vi "AB_RW_Project_Source_Library.vi"(7 "action":T3, 8 "error in (no error)":errorcluster, 9 "index in":i32, 10 "dataSource in":T2, 11 "buildObject":T1) -> (0 "error out":errorcluster, 1 "index out":i32, 2 "dataSource out":T2, 3 "buildObject out":T1)   [LabVIEW 2020]
doc: "Reads and writes the data to the object property bag."
uses:
  <resource>/Framework/Providers/API/ItemRef.ctl
  <vilib>/AppBuilder/RW_Project/AB_RW_Project_Source_Library_Data.ctl
  <vilib>/AppBuilder/RW_Project/AB_RW_Project_PropBag_Action.ctl
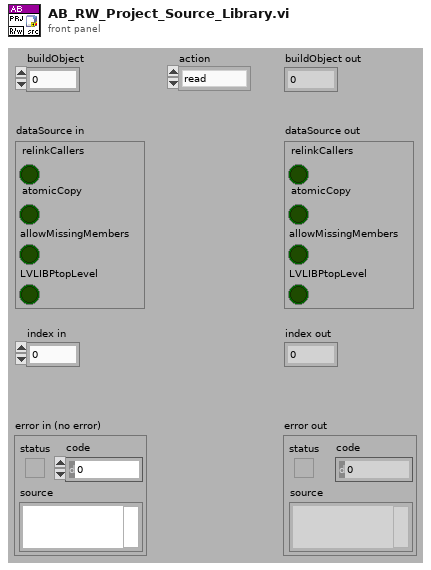
[diagram p1: front panel]
types:
  T1 = typedef "ItemRef.ctl" = u64
  T2 = typedef "AB_RW_Project_Source_Library_Data.ctl" = cluster{"relinkCallers":bool, "atomicCopy":bool, "allowMissingMembers":bool, "LVLIBPtopLevel":bool}
  T3 = typedef "AB_RW_Project_PropBag_Action.ctl" = enum16{"read", "write", "clear", "readPrevious", "writePrevious", "clearPrevious"}
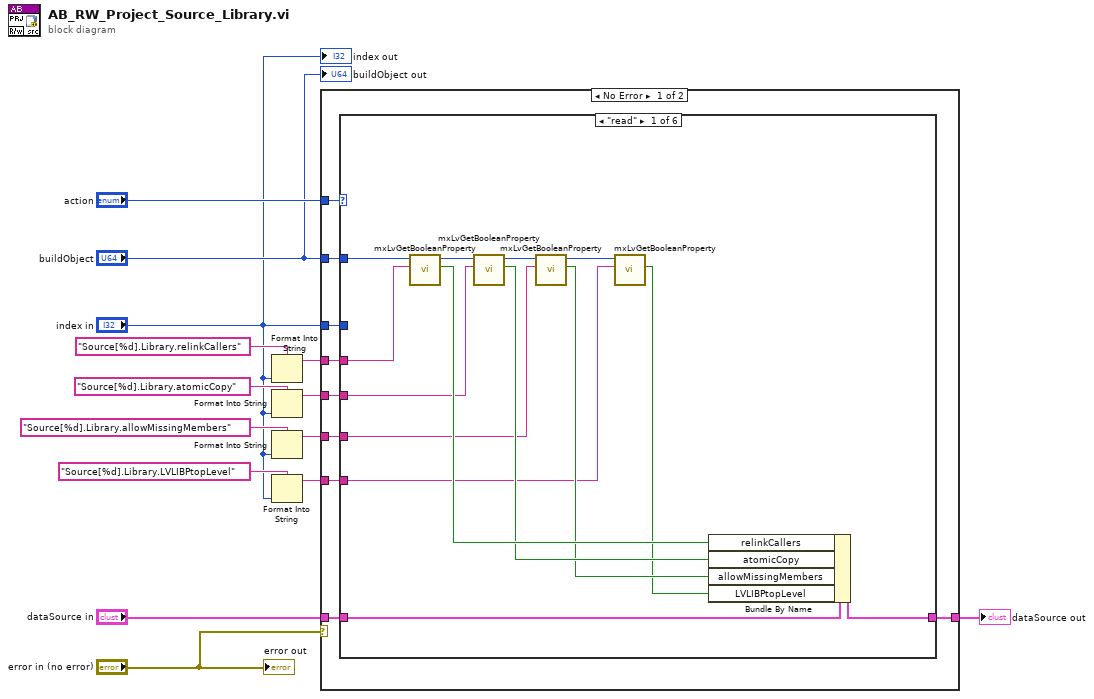
[diagram p0: block diagram]
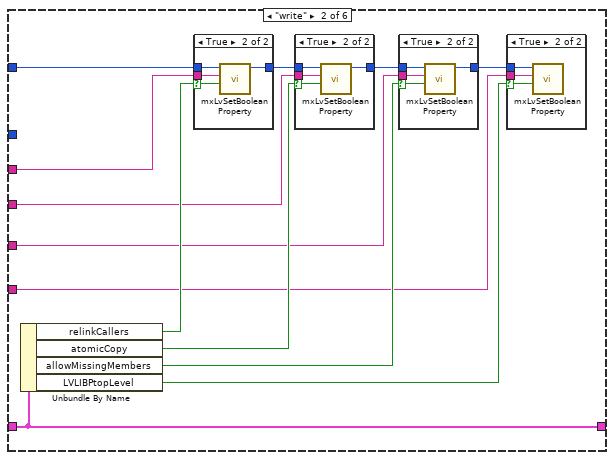
[diagram p2: hidden frame]
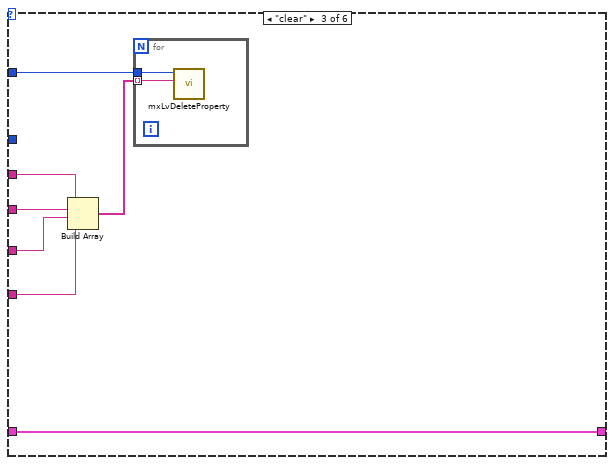
[diagram p7: hidden frame]
diagram:
  n1 = Format Into String(format string="Source[%d].Library.relinkCallers", "index in") -> (resulting string=w11:string)  [unwired: 2 in, 1 out]
  n2 = Format Into String(format string="Source[%d].Library.atomicCopy", "index in") -> (resulting string=w9:string)  [unwired: 2 in, 1 out]
  n3 = Format Into String(format string="Source[%d].Library.allowMissingMembers", "index in") -> (resulting string=w4:string)  [unwired: 2 in, 1 out]
  n4 = Format Into String(format string="Source[%d].Library.LVLIBPtopLevel", "index in") -> (resulting string=w1:string)  [unwired: 2 in, 1 out]
  n5 = case shown="No Error" "error in (no error)" {
    tunnel: "action" -> [w23 _]
    tunnel: "dataSource in" -> [w22 w81]
    tunnel: w11 -> [w21 _]
    tunnel: w9 -> [w20 _]
    tunnel: "index in" -> [w19 _]
    tunnel: [w18 w81] -> w8
    tunnel: "buildObject" -> [w17 _]
    tunnel: w4 -> [w16 _]
    tunnel: w1 -> [w15 _]
    frame No Error {
      n6 = case shown="\"read\"" w23 {
        tunnel: w17 -> [w35 w49 w71 _ _ _]
        tunnel: w22 -> [w37 w50 w75 w78 w79 w80]
        tunnel: w21 -> [w33 w47 w74 _ _ _]
        tunnel: w20 -> [w31 w45 w73 _ _ _]
        tunnel: w19 -> [_ _ _ _ _ _]
        tunnel: [w36 w50 w75 w78 w79 w80] -> w18
        tunnel: w16 -> [w29 w42 w70 _ _ _]
        tunnel: w15 -> [w25 w39 w69 _ _ _]
        frame "read" {
          n7 = call <resource>:"mxLvGetBooleanProperty.vi"("Tag"=w33, "Item"=w35) -> ("Value"=w34:bool, "Item"=w32:T1)  [unwired: 7 in, 1 out]
          n8 = call <resource>:"mxLvGetBooleanProperty.vi"("Tag"=w31, "Item"=w32) -> ("Value"=w30:bool, "Item"=w28:T1)  [unwired: 7 in, 1 out]
          n9 = call <resource>:"mxLvGetBooleanProperty.vi"("Tag"=w29, "Item"=w28) -> ("Value"=w27:bool, "Item"=w26:T1)  [unwired: 7 in, 1 out]
          n10 = call <resource>:"mxLvGetBooleanProperty.vi"("Tag"=w25, "Item"=w26) -> ("Value"=w24:bool)  [unwired: 7 in, 2 out]
          n11 = Bundle By Name(cluster=w37, "relinkCallers"=w34, "atomicCopy"=w30, "allowMissingMembers"=w27, "LVLIBPtopLevel"=w24) -> (w36:T2)
        }
        frame "write" {
          n12 = Unbundle By Name(w50) -> ("relinkCallers"=w46:bool, "atomicCopy"=w44:bool, "allowMissingMembers"=w43:bool, "LVLIBPtopLevel"=w38:bool)
          n13 = case shown="True" w46 {
            selector: w46 -> [_ w66]
            tunnel: w49 -> [w64 w68]
            tunnel: w47 -> [_ w67]
            tunnel: [w64 w65] -> w48
            frame False {
            }
            frame True {
              n14 = call <resource>:"mxLvSetBooleanProperty.vi"("Value (F)"=w66, "Tag"=w67, "Item"=w68) -> ("Item"=w65:T1)  [unwired: 7 in, 1 out]
            }
          }
          n15 = case shown="True" w44 {
            selector: w44 -> [_ w61]
            tunnel: w48 -> [w59 w63]
            tunnel: w45 -> [_ w62]
            tunnel: [w59 w60] -> w41
            frame False {
            }
            frame True {
              n16 = call <resource>:"mxLvSetBooleanProperty.vi"("Value (F)"=w61, "Tag"=w62, "Item"=w63) -> ("Item"=w60:T1)  [unwired: 7 in, 1 out]
            }
          }
          n17 = case shown="True" w43 {
            selector: w43 -> [_ w56]
            tunnel: w41 -> [w54 w58]
            tunnel: w42 -> [_ w57]
            tunnel: [w54 w55] -> w40
            frame False {
            }
            frame True {
              n18 = call <resource>:"mxLvSetBooleanProperty.vi"("Value (F)"=w56, "Tag"=w57, "Item"=w58) -> ("Item"=w55:T1)  [unwired: 7 in, 1 out]
            }
          }
          n19 = case shown="True" w38 {
            selector: w38 -> [_ w51]
            tunnel: w40 -> [_ w53]
            tunnel: w39 -> [_ w52]
            frame False {
            }
            frame True {
              n20 = call <resource>:"mxLvSetBooleanProperty.vi"("Value (F)"=w51, "Tag"=w52, "Item"=w53) -> ()  [unwired: 7 in, 2 out]
            }
          }
        }
        frame "clear" {
          n21 = Build Array(w74, w73, w70, w69) -> (w72:string[])
          n22 = for {
            tunnel: w71 -> [w77]
            tunnel: w72 -> [w76] mode=indexing
            n23 = call <resource>:"mxLvDeleteProperty.vi"("Tag"=w76, "Item"=w77) -> ()  [unwired: 8 in, 2 out]
          }
        }
        frame "readPrevious" {
        }
        frame "writePrevious" {
        }
        frame "clearPrevious" {
        }
      }
    }
    frame Error {
    }
  }
  "dataSource out" <- w8
  "error out" <- "error in (no error)"
  "buildObject out" <- "buildObject"
  "index out" <- "index in"
